vi "Go to zero.vi"(5 "Starting angle M1":dbl, 7 "Starting angle M2":dbl, 8 "error in (no error)":errorcluster, 11 "VISA resource name":refnum<visa-resource-name>) -> (0 "error out":errorcluster)   [LabVIEW 2020]
uses:
  Public/Controls/Move motor parameters--cluster.ctl
  Public/Controls/Motor direction.ctl
  Public/Controls/Step style.ctl
  Public/Write--move.vi
  Control de MaP.lvlib
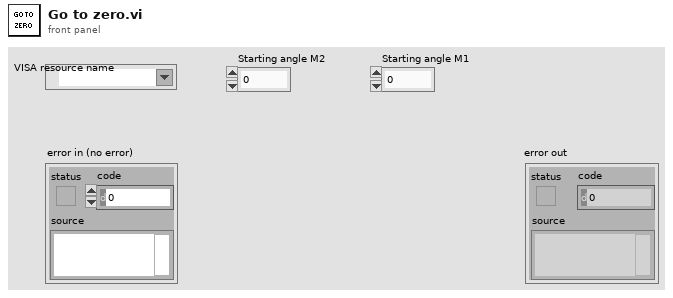
[diagram p1: front panel]
types:
  T1 = typedef "Control de MaP.lvlib/Move motor parameters--cluster.ctl" = cluster{"Action":u8, "Direction motor 1":T2, "Direction motor 2":T2, "Steps motor 1":u16, "Steps motor 2":u16, "Step style motor 1":T3, "Step style motor 2":T3}
  T2 = typedef "Control de MaP.lvlib/Motor direction.ctl" = u8
  T3 = typedef "Control de MaP.lvlib/Step style.ctl" = u8
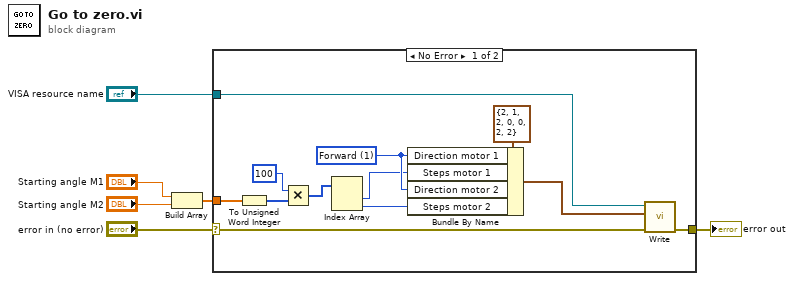
[diagram p0: block diagram]
diagram:
  n1 = Build Array("Starting angle M1", "Starting angle M2") -> (w1:dbl[])
  n2 = case shown="No Error" "error in (no error)" {
    selector: "error in (no error)" -> [w15 w19]
    tunnel: "VISA resource name" -> [w16 _]
    tunnel: w1 -> [w11 _]
    tunnel: [w7 w19] -> w4
    frame No Error {
      w14 = T2 1 items=["", "Forward", "Backward"] ("Direction motor 1")
      n3 = To Unsigned Word Integer(number=w11) -> (unsigned 16bit integer=w13:u16[])
      n4 = Multiply(x=u16 100 ("y"), y=w13) -> (x*y=w10:u16[])
      n5 = Index Array(array=w10) -> (element #1=w9:u16, element #2=w8:u16)  [unwired: 2 in]
      n6 = Bundle By Name(cluster=T1 {"Action"=2, "Direction motor 1"=1, "Direction motor 2"=2, "Steps motor 1"=0, "Steps motor 2"=0, "Step style motor 1"=2, "Step style motor 2"=2} ("Comando"), "Direction motor 1"=w14, "Steps motor 1"=w9, "Direction motor 2"=w14, "Steps motor 2"=w8) -> (w18:T1)
      n7 = call-poly "Write.vi"("error in (no error)"=w15, "Comando"=w18, "VISA resource name"=w16) -> ("error out"=w7:errorcluster)  [unwired: 6 in, 2 out]
    }
    frame Error {
    }
  }
  "error out" <- w4
